vi "Translator.Translate.Controls.vi"(7 "group":string, 8 "error in":errorcluster, 9 "font name":string, 10 "Controls out":T1[](array[typedef]), 11 "Translation file":path=path "D:/PL_0125_Sapphire_Automation_branches/SOFTWARE_v1.1-Translation/settings/Translation-Chinese.ini") -> (0 "error out":errorcluster)   [LabVIEW 2019, in "Tools.lvlib"]
uses:
  Tools.lvlib
  Translator.ControlData.ctl
  Translator.ControlTypes.ctl
  <vilib>/Utility/miscctls.llb/LVRowAndColumnTypeDef.ctl
  Translator.File.MatchStrings (Single).vi
  Translator.File.MatchStrings (Array).vi
  <vilib>/Utility/config.llb/NI_LVConfig.lvlib
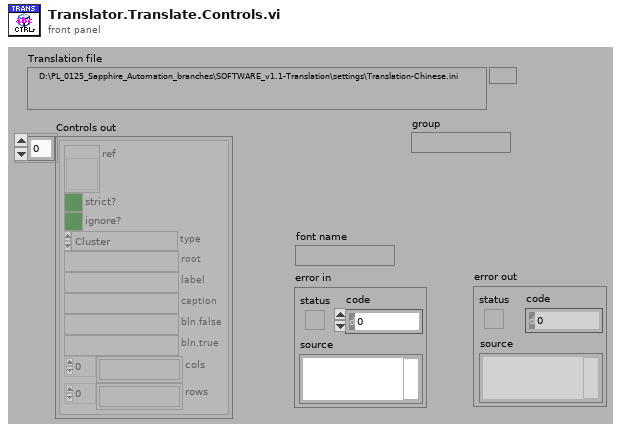
[diagram p1: front panel]
types:
  T1 = typedef "Tools.lvlib/Translator.ControlData.ctl" = cluster{"ref":refnum<vi>, "strict?":bool, "ignore?":bool, "type":T2, "root":string, "label":string, "caption":string, "bln.false":string, "bln.true":string, "cols":string[], "rows":string[]}
  T2 = typedef "Tools.lvlib/Translator.ControlTypes.ctl" = enum16{"Cluster", "Array", "Boolean", "Ring", "String", "Tab", "Listbox", "Multicolumn listbox", "Table", "Other"}
  T3 = typedef "LVRowAndColumnTypeDef.ctl" = cluster{"Row":i32, "Column":i32}
  T4 = typedef "NI_LVConfig.lvlib/Config Data RefNum.ctl" = refnum<k1>
  T5 = typedef "LVBoundsTypeDef.ctl" = cluster{"Width":u32, "Height":u32}
  T6 = typedef "LVPositionTypeDef.ctl" = cluster{"Left":i32, "Top":i32}
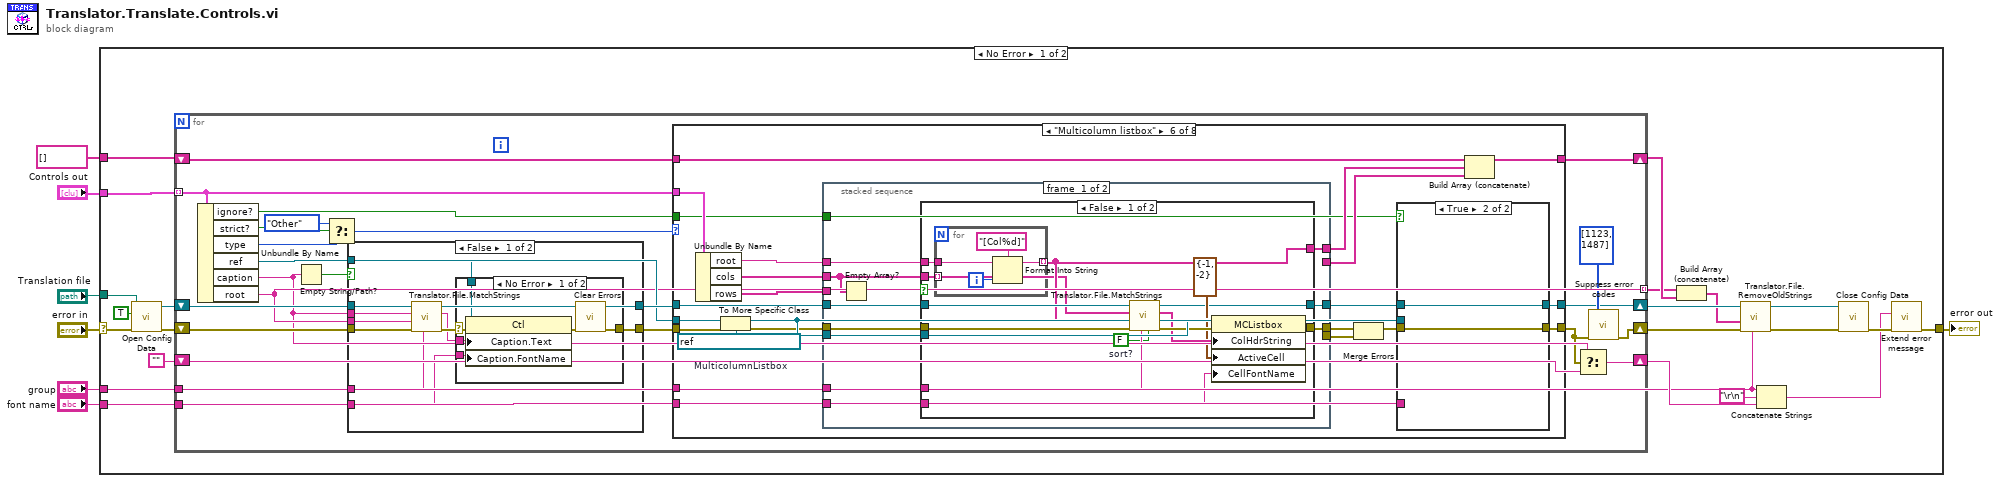
[diagram p0: block diagram]
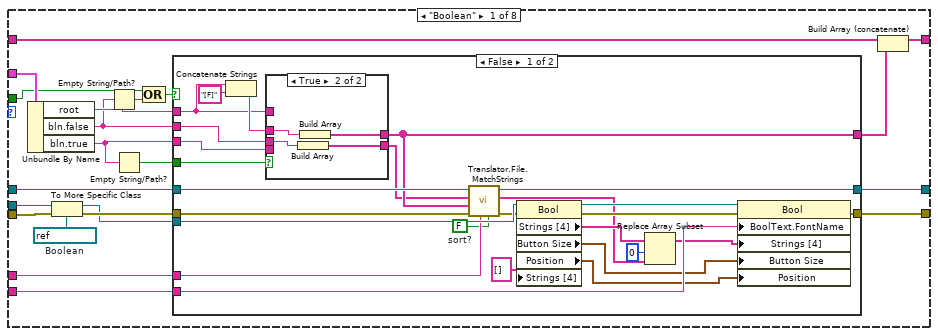
[diagram p4: hidden frame]
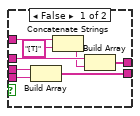
[diagram p5: hidden frame]
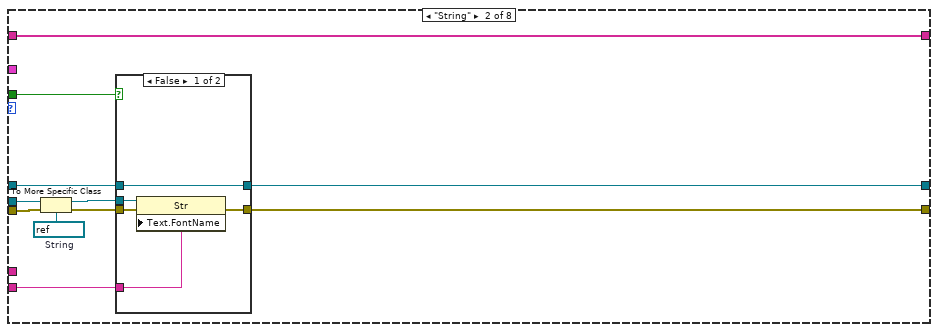
[diagram p7: hidden frame]
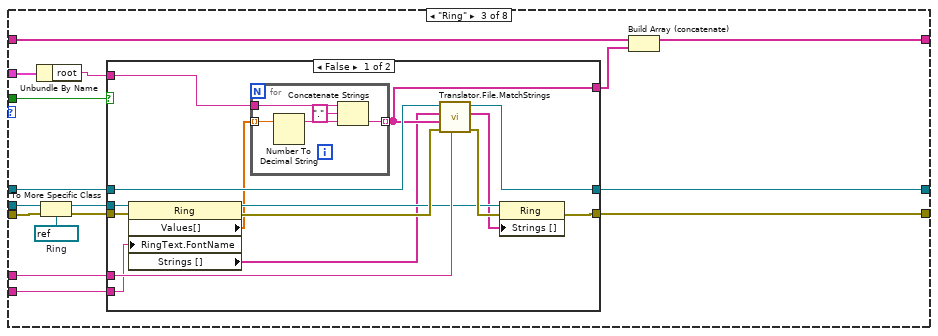
[diagram p9: hidden frame]
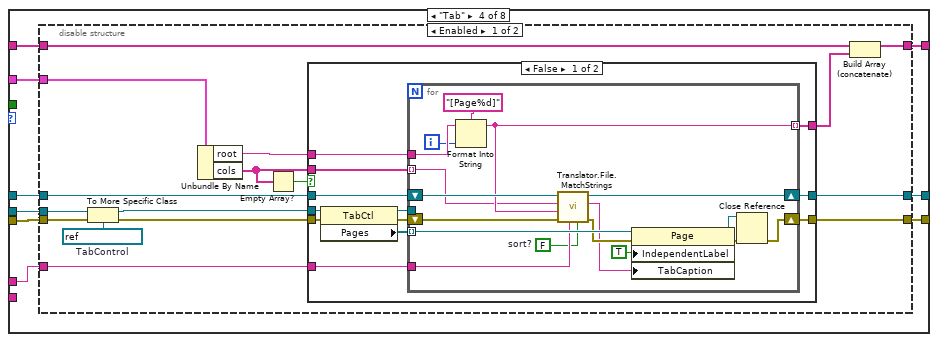
[diagram p11: hidden frame]
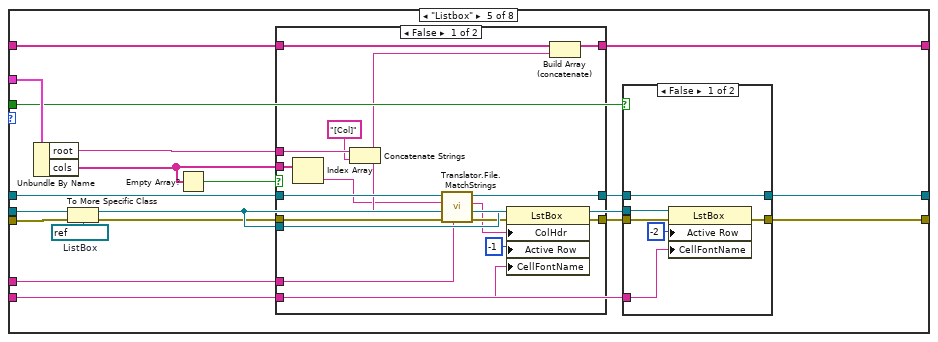
[diagram p14: hidden frame]
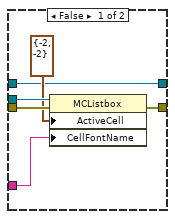
[diagram p17: hidden frame]
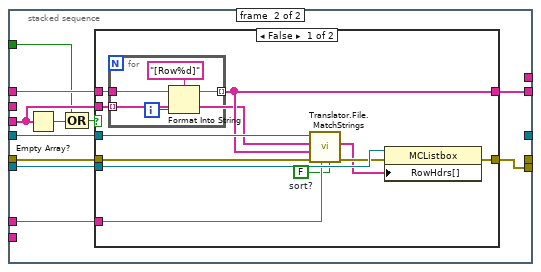
[diagram p19: hidden frame]
diagram:
  n1 = case shown="No Error" "error in" {
    selector: "error in" -> [w17 w477]
    tunnel: "Controls out" -> [w22 _]
    tunnel: [w15 w477] -> w5
    tunnel: "Translation file" -> [w11 _]
    tunnel: "group" -> [w10 _]
    tunnel: "font name" -> [w29 _]
    tunnel: string[] [] -> [w26 _]
    frame No Error {
      n2 = call <vilib>:"Open Config Data.vi"("error in (no error)"=w17, "create file if necessary (T)"=TRUE, "configuration file path"=w11) -> ("error out"=w8:errorcluster, "refnum"=w9:T4)  [unwired: 6 in, 1 out]
      n3 = for {
        tunnel: w22 -> [w53] mode=indexing
        tunnel: w10 -> [w50]
        shift-right: [w30] -> w28
        shift-left: w9 -> [w51]
        tunnel: w29 -> [w31]
        shift-right: [w40] -> w25
        shift-left: w26 -> [w41]
        tunnel: [w39] -> w24 mode=indexing
        shift-right: [w35] -> w20
        shift-left: "" -> [w37]
        shift-right: [w33] -> w27
        shift-left: w8 -> [w52]
        n4 = Unbundle By Name(w53) -> ("ignore?"=w38:bool, "strict?"=w45:bool, "type"=w44:T2, "ref"=w46:refnum<vi>, "caption"=w36:string, "root"=w39:string)
        n5 = Empty String/Path?(string/path=w36) -> (empty?=w47:bool)
        n6 = Select(t=Translator.ControlTypes."Other", s=w45, f=w44) -> (s? t:f=w42:T2)
        n7 = case shown="False" w47 {
          tunnel: w52 -> [w55 w72]
          tunnel: w51 -> [w63 w71]
          tunnel: w50 -> [w56 _]
          tunnel: [w62 w71] -> w49
          tunnel: [w61 w72] -> w48
          tunnel: w46 -> [w60 _]
          tunnel: w31 -> [w58 _]
          tunnel: w36 -> [w54 _]
          tunnel: w39 -> [w57 _]
          frame False {
            n8 = call-poly "Translator.File.MatchStrings.vi"("group"=w56, "error in"=w55, "label"=w57, "default value"=w54, "refnum in"=w63) -> ("error out"=w61:errorcluster, "value out"=w59:string, "refnum out"=w62:T4)  [unwired: 3 in, 1 out]
            n9 = case shown="No Error" w61 {
              selector: w61 -> [w69 w70]
              tunnel: [w65 w70] -> _
              tunnel: w60 -> [w67 _]
              tunnel: w58 -> [w66 _]
              tunnel: w59 -> [w64 _]
              frame No Error {
                n10 = property class="Ctl"(reference=w67, error in=w69, "Caption.Text"=w64, "Caption.FontName"=w66) -> (error out=w68:errorcluster)  [unwired: 1 out]
                n11 = call <vilib>:"Clear Errors.vi"("error in (no error)"=w68) -> ("error out"=w65:errorcluster)  [unwired: 5 in, 1 out]
              }
              frame Error {
              }
            }
          }
          frame True {
          }
        }
        n12 = case shown="\"Multicolumn listbox\"" w42 {
          tunnel: w46 -> [w91 w142 w165 w197 w261 w308 w397 _]
          tunnel: w48 -> [w92 w143 w166 w198 w262 w309 w398 w476]
          tunnel: w53 -> [w90 _ w154 w191 w266 w316 w405 _]
          tunnel: [w76 w138 w161 w196 w256 w305 w395 w476] -> w34
          tunnel: w49 -> [w88 w134 w158 w195 w264 w314 w403 w474]
          tunnel: w50 -> [w89 _ w157 w194 w263 w312 w401 _]
          tunnel: w31 -> [w74 w139 w162 _ w250 w297 w386 _]
          tunnel: w41 -> [w84 w137 w160 w193 w254 w301 w392 w475]
          tunnel: [w86 w137 w155 w192 w253 w302 w389 w475] -> w40
          tunnel: w38 -> [w75 w136 w159 _ w252 w298 w387 _]
          tunnel: [w73 w135 w156 w190 w249 w296 w385 w474] -> w30
          frame "Boolean" {
            w93 = refnum<vi> refnum  # Boolean
            n13 = Unbundle By Name(w90) -> ("root"=w87:string, "bln.false"=w83:string, "bln.true"=w82:string)
            n14 = To More Specific Class(target class=w93, reference=w91, error in=w92) -> (specific class reference=w77:refnum<vi>, error out=w80:errorcluster)
            n15 = Empty String/Path?(string/path=w83) -> (empty?=w79:bool)
            n16 = Empty String/Path?(string/path=w82) -> (empty?=w81:bool)
            n17 = Compound Arithmetic op=OR(w75, w79) -> (w78:bool)
            n18 = case shown="False" w78 {
              tunnel: w77 -> [w113 _]
              tunnel: w80 -> [w98 w133]
              tunnel: [w119 w133] -> w76
              tunnel: w87 -> [w108 _]
              tunnel: w89 -> [w99 _]
              tunnel: w88 -> [w111 w132]
              tunnel: [w100 _] -> w85
              tunnel: w82 -> [w106 _]
              tunnel: w83 -> [w107 _]
              tunnel: w81 -> [w110 _]
              tunnel: w74 -> [w105 _]
              tunnel: [w95 w132] -> w73
              frame False {
                w94 = FALSE  # sort?
                n19 = Concatenate Strings(w108, "[F]" ("format string")) -> (w109:string)
                n20 = case shown="True" w110 {
                  tunnel: w108 -> [w126 _]
                  tunnel: [w125 w130] -> w100
                  tunnel: w109 -> [w124 w131]
                  tunnel: w107 -> [w122 w129]
                  tunnel: w106 -> [w121 _]
                  tunnel: [w120 w128] -> w97
                  frame False {
                    n21 = Build Array(w122, w121) -> (w120:string[])
                    n22 = Concatenate Strings(w126, "[T]" ("format string")) -> (w123:string)
                    n23 = Build Array(w124, w123) -> (w125:string[])
                  }
                  frame True {
                    n24 = Build Array(w129) -> (w128:string[])
                    n25 = Build Array(w131) -> (w130:string[])
                  }
                }
                n26 = call-poly "Translator.File.MatchStrings.vi"("sort? (T)"=w94, "group"=w99, "error in"=w98, "labels"=w100, "default values"=w97, "refnum in"=w111) -> ("error out"=w112:errorcluster, "values out"=w102:string[], "refnum out"=w95:T4)  [unwired: 2 in, 1 out]
                n27 = property class="Bool"(reference=w113, error in=w112, "Strings [4]"=string[] []) -> (reference out=w115:refnum<vi>, error out=w116:errorcluster, "Strings [4]"=w118:string[], "Button Size"=w103:T5, "Position"=w101:T6)
                n28 = Replace Array Subset(array=w118, new element=w102, index=0) -> (w104:string[])
                n29 = property class="Bool"(reference=w115, error in=w116, "BoolText.FontName"=w105, "Strings [4]"=w104, "Button Size"=w103, "Position"=w101) -> (error out=w119:errorcluster)  [unwired: 1 out]
              }
              frame True {
              }
            }
            n30 = Build Array (concatenate)(w84, w85) -> (w86:string[])
          }
          frame "String" {
            w144 = refnum<vi> refnum  # String
            n31 = To More Specific Class(target class=w144, reference=w142, error in=w143) -> (specific class reference=w141:refnum<vi>, error out=w140:errorcluster)
            n32 = case shown="False" w136 {
              tunnel: w141 -> [w149 _]
              tunnel: w140 -> [w148 w151]
              tunnel: w139 -> [w146 _]
              tunnel: [w147 w151] -> w138
              tunnel: [w145 w150] -> w135
              tunnel: w134 -> [w145 w150]
              frame False {
                n33 = property class="Str"(reference=w149, error in=w148, "Text.FontName"=w146) -> (error out=w147:errorcluster)  [unwired: 1 out]
              }
              frame True {
              }
            }
          }
          frame "Ring" {
            w167 = refnum<vi> refnum  # Ring
            n34 = Unbundle By Name(w154) -> ("root"=w153:string)
            n35 = To More Specific Class(target class=w167, reference=w165, error in=w166) -> (specific class reference=w164:refnum<vi>, error out=w163:errorcluster)
            n36 = case shown="False" w159 {
              tunnel: w164 -> [w182 _]
              tunnel: w163 -> [w181 w189]
              tunnel: w162 -> [w172 _]
              tunnel: [w176 w189] -> w161
              tunnel: w158 -> [w179 w188]
              tunnel: w157 -> [w178 _]
              tunnel: [w173 w188] -> w156
              tunnel: w153 -> [w170 _]
              tunnel: [w169 _] -> w152
              frame False {
                n37 = property class="Ring"(reference=w182, error in=w181, "RingText.FontName"=w172) -> (reference out=w175:refnum<vi>, error out=w180:errorcluster, "Values[]"=w171:ext[], "Strings []"=w168:string[])
                n38 = for {
                  tunnel: w171 -> [w184] mode=indexing
                  tunnel: [w186] -> w169 mode=indexing
                  tunnel: w170 -> [w185]
                  n39 = Number To Decimal String(number=w184) -> (decimal integer string=w183:string)  [unwired: 1 in]
                  n40 = Concatenate Strings(w185, "." ("string"), w183) -> (w186:string)
                }
                n41 = call-poly "Translator.File.MatchStrings.vi"("group"=w178, "error in"=w180, "labels"=w169, "default values"=w168, "refnum in"=w179) -> ("error out"=w177:errorcluster, "values out"=w174:string[], "refnum out"=w173:T4)  [unwired: 3 in, 1 out]
                n42 = property class="Ring"(reference=w175, error in=w177, "Strings []"=w174) -> (error out=w176:errorcluster)  [unwired: 1 out]
              }
              frame True {
              }
            }
            n43 = Build Array (concatenate)(w160, w152) -> (w155:string[])
          }
          frame "Tab" {
            n44 = disable-structure shown="Enabled" {
              disable-tunnel: w198 -> [w214 w246]
              disable-tunnel: w197 -> [w213 _]
              disable-tunnel: [w212 w246] -> w196
              disable-tunnel: w195 -> [w211 _]
              disable-tunnel: w194 -> [w210 _]
              disable-tunnel: w193 -> [w209 w247]
              disable-tunnel: [w208 w247] -> w192
              disable-tunnel: w191 -> [w200 _]
              disable-tunnel: [w199 _] -> w190
              frame Enabled {
                w205 = refnum<vi> refnum  # TabControl
                n45 = To More Specific Class(target class=w205, reference=w213, error in=w214) -> (specific class reference=w206:refnum<vi>, error out=w207:errorcluster)
                n46 = Unbundle By Name(w200) -> ("root"=w204:string, "cols"=w203:string[])
                n47 = Empty Array?(array=w203) -> (empty?=w202:bool)
                n48 = case shown="False" w202 {
                  tunnel: w207 -> [w225 w245]
                  tunnel: w206 -> [w222 _]
                  tunnel: [w221 w245] -> w212
                  tunnel: w211 -> [w220 w244]
                  tunnel: w204 -> [w219 _]
                  tunnel: w203 -> [w218 _]
                  tunnel: w210 -> [w217 _]
                  tunnel: [w216 _] -> w201
                  tunnel: [w215 w244] -> w199
                  frame False {
                    n49 = property class="TabCtl"(reference=w222, error in=w225) -> (reference out=w223:refnum<vi>, error out=w224:errorcluster, "Pages"=w226:refnum<vi>[])
                    n50 = for {
                      tunnel: w226 -> [w243] mode=indexing
                      tunnel: w223 -> [_]
                      shift-right: [w239] -> w221
                      shift-left: w224 -> [w229]
                      tunnel: w218 -> [w230] mode=indexing
                      tunnel: w219 -> [w238]
                      tunnel: w217 -> [w232]
                      tunnel: [w231] -> w216 mode=indexing
                      shift-right: [w228] -> w215
                      shift-left: w220 -> [w241]
                      i -> [w236]
                      w227 = FALSE  # sort?
                      n51 = Format Into String(format string="[Page%d]", initial string=w238, w236) -> (resulting string=w231:string)  [unwired: 1 in, 1 out]
                      n52 = call-poly "Translator.File.MatchStrings.vi"("sort? (F)"=w227, "group"=w232, "error in"=w229, "label"=w231, "default value"=w230, "refnum in"=w241) -> ("error out"=w242:errorcluster, "value out"=w235:string, "refnum out"=w228:T4)  [unwired: 2 in, 1 out]
                      n53 = property class="Page"(reference=w243, error in=w242, "IndependentLabel"=TRUE ("Independent Label"), "TabCaption"=w235) -> (reference out=w234:refnum<vi>, error out=w240:errorcluster)
                      n54 = Close Reference(reference=w234, error in (no error)=w240) -> (error out=w239:errorcluster)
                    }
                  }
                  frame True {
                  }
                }
                n55 = Build Array (concatenate)(w209, w201) -> (w208:string[])
              }
              frame Disabled {
              }
            }
          }
          frame "Listbox" {
            w260 = refnum<vi> refnum  # ListBox
            n56 = Unbundle By Name(w266) -> ("root"=w265:string, "cols"=w259:string[])
            n57 = To More Specific Class(target class=w260, reference=w261, error in=w262) -> (specific class reference=w258:refnum<vi>, error out=w255:errorcluster)
            n58 = Empty Array?(array=w259) -> (empty?=w251:bool)
            n59 = case shown="False" w251 {
              tunnel: [w291 w294] -> w257
              tunnel: w255 -> [w276 w294]
              tunnel: w265 -> [w290 _]
              tunnel: w259 -> [w285 _]
              tunnel: w264 -> [w289 w292]
              tunnel: w263 -> [w278 _]
              tunnel: w258 -> [w288 _]
              tunnel: w254 -> [w283 w293]
              tunnel: [w282 w293] -> w253
              tunnel: w250 -> [w280 _]
              tunnel: [w275 w292] -> w248
              frame False {
                n60 = Index Array(array=w285) -> (element=w277:string)  [unwired: 1 in]
                n61 = Concatenate Strings(w290, "[Col]" ("format string")) -> (w279:string)
                n62 = call-poly "Translator.File.MatchStrings.vi"("group"=w278, "error in"=w276, "label"=w279, "default value"=w277, "refnum in"=w289) -> ("error out"=w287:errorcluster, "value out"=w284:string, "refnum out"=w275:T4)  [unwired: 3 in, 1 out]
                n63 = property class="LstBox"(reference=w288, error in=w287, "ColHdr"=w284, "Active Row"=-1 ("Active Row:Active Row Number"), "CellFontName"=w280) -> (error out=w291:errorcluster)  [unwired: 1 out]
                n64 = Build Array (concatenate)(w283, w279) -> (w282:string[])
              }
              frame True {
              }
            }
            n65 = case shown="False" w252 {
              tunnel: w258 -> [w272 _]
              tunnel: w257 -> [w271 w274]
              tunnel: w250 -> [w269 _]
              tunnel: [w268 w274] -> w256
              tunnel: [w267 w273] -> w249
              tunnel: w248 -> [w267 w273]
              frame False {
                n66 = property class="LstBox"(reference=w272, error in=w271, "Active Row"=-2 ("Active Row:Active Row Number"), "CellFontName"=w269) -> (error out=w268:errorcluster)  [unwired: 1 out]
              }
              frame True {
              }
            }
          }
          frame "Multicolumn listbox" {
            w307 = refnum<vi> refnum  # MulticolumnListbox
            n67 = Unbundle By Name(w316) -> ("root"=w315:string, "cols"=w313:string[], "rows"=w311:string[])
            n68 = To More Specific Class(target class=w307, reference=w308, error in=w309) -> (specific class reference=w304:refnum<vi>, error out=w303:errorcluster)
            n69 = stacked-sequence {
              tunnel: [w330 _] -> w317
              tunnel: w303 -> [w336 w367]
              tunnel: w315 -> [w335 w366]
              tunnel: w314 -> [w334 w365]
              tunnel: w313 -> [w331 _]
              tunnel: w312 -> [w333 w364]
              tunnel: w311 -> [_ w363]
              tunnel: [_ w360] -> w310
              tunnel: w304 -> [w332 w362]
              tunnel: [w329 _] -> w300
              tunnel: [_ w361] -> w299
              tunnel: w298 -> [_ w357]
              tunnel: w297 -> [w328 _]
              tunnel: [w326 _] -> w295
              frame #0 {
                n70 = Empty Array?(array=w331) -> (empty?=w327:bool)
                n71 = case shown="False" w327 {
                  tunnel: [w350 w356] -> w330
                  tunnel: w336 -> [w340 w356]
                  tunnel: w335 -> [w349 _]
                  tunnel: w331 -> [w339 _]
                  tunnel: w334 -> [w348 w355]
                  tunnel: w333 -> [w342 _]
                  tunnel: w332 -> [w347 _]
                  tunnel: [w341 _] -> w329
                  tunnel: w328 -> [w343 _]
                  tunnel: [w338 w355] -> w326
                  frame False {
                    w337 = FALSE  # sort?
                    n72 = for {
                      tunnel: w349 -> [w353]
                      tunnel: [w351] -> w341 mode=indexing
                      tunnel: w339 -> [_] mode=indexing
                      i -> [w352]
                      n73 = Format Into String(format string="[Col%d]", initial string=w353, w352) -> (resulting string=w351:string)  [unwired: 1 in, 1 out]
                    }
                    n74 = call-poly "Translator.File.MatchStrings.vi"("sort? (T)"=w337, "group"=w342, "error in"=w340, "labels"=w341, "default values"=w339, "refnum in"=w348) -> ("error out"=w346:errorcluster, "values out"=w345:string[], "refnum out"=w338:T4)  [unwired: 2 in, 1 out]
                    n75 = property class="MCListbox"(reference=w347, error in=w346, "ColHdrString"=w345, "ActiveCell"=T3 {"Row"=-1, "Column"=-2} ("Active Cell:Active Cell"), "CellFontName"=w343) -> (error out=w350:errorcluster)  [unwired: 1 out]
                  }
                  frame True {
                  }
                }
              }
              frame #1 {
                n76 = Empty Array?(array=w363) -> (empty?=w359:bool)
                n77 = Compound Arithmetic op=OR(w357, w359) -> (w358:bool)
                n78 = case shown="False" w358 {
                  tunnel: [w378 w383] -> w360
                  tunnel: w367 -> [w369 w383]
                  tunnel: w366 -> [w377 _]
                  tunnel: w363 -> [w370 _]
                  tunnel: w365 -> [w376 _]
                  tunnel: w364 -> [w372 _]
                  tunnel: w362 -> [w375 _]
                  tunnel: [w371 _] -> w361
                  frame False {
                    w368 = FALSE  # sort?
                    n79 = for {
                      tunnel: w377 -> [w381]
                      tunnel: [w379] -> w371 mode=indexing
                      tunnel: w370 -> [_] mode=indexing
                      i -> [w380]
                      n80 = Format Into String(format string="[Row%d]", initial string=w381, w380) -> (resulting string=w379:string)  [unwired: 1 in, 1 out]
                    }
                    n81 = call-poly "Translator.File.MatchStrings.vi"("sort? (T)"=w368, "group"=w372, "error in"=w369, "labels"=w371, "default values"=w370, "refnum in"=w376) -> ("error out"=w374:errorcluster, "values out"=w373:string[])  [unwired: 2 in, 2 out]
                    n82 = property class="MCListbox"(reference=w375, error in=w374, "RowHdrs[]"=w373) -> (error out=w378:errorcluster)  [unwired: 1 out]
                  }
                  frame True {
                  }
                }
              }
            }
            n83 = Merge Errors(w317, w310) -> (w306:errorcluster)
            n84 = case shown="True" w298 {
              tunnel: w306 -> [w323 w325]
              tunnel: [w322 w325] -> w305
              tunnel: w304 -> [w321 _]
              tunnel: w297 -> [w319 _]
              tunnel: [w318 w324] -> w296
              tunnel: w295 -> [w318 w324]
              frame False {
                n85 = property class="MCListbox"(reference=w321, error in=w323, "ActiveCell"=T3 {"Row"=-2, "Column"=-2} ("Active Cell:Active Cell"), "CellFontName"=w319) -> (error out=w322:errorcluster)  [unwired: 1 out]
              }
              frame True {
              }
            }
            n86 = Build Array (concatenate)(w301, w300, w299) -> (w302:string[])
          }
          frame "Table" {
            w394 = refnum<vi> refnum  # Table
            n87 = Unbundle By Name(w405) -> ("root"=w404:string, "cols"=w402:string[], "rows"=w400:string[])
            n88 = To More Specific Class(target class=w394, reference=w397, error in=w398) -> (specific class reference=w388:refnum<vi>, error out=w393:errorcluster)
            n89 = stacked-sequence {
              tunnel: [w418 _] -> w406
              tunnel: w393 -> [w424 w454]
              tunnel: w404 -> [w423 w453]
              tunnel: w403 -> [w422 w452]
              tunnel: w402 -> [w419 _]
              tunnel: w401 -> [w421 w451]
              tunnel: w400 -> [_ w450]
              tunnel: [_ w448] -> w399
              tunnel: w388 -> [w420 w449]
              tunnel: [_ w447] -> w391
              tunnel: [w417 _] -> w390
              tunnel: w387 -> [_ w444]
              tunnel: w386 -> [w415 _]
              tunnel: [_ w443] -> w384
              frame #0 {
                n90 = Empty Array?(array=w419) -> (empty?=w416:bool)
                n91 = case shown="False" w416 {
                  tunnel: [w437 w442] -> w418
                  tunnel: w424 -> [w426 w442]
                  tunnel: w423 -> [w436 _]
                  tunnel: w419 -> [w427 _]
                  tunnel: w422 -> [w435 _]
                  tunnel: w421 -> [w429 _]
                  tunnel: w420 -> [w434 _]
                  tunnel: [w428 _] -> w417
                  tunnel: w415 -> [w430 _]
                  frame False {
                    w425 = FALSE  # sort?
                    n92 = for {
                      tunnel: w436 -> [w440]
                      tunnel: [w438] -> w428 mode=indexing
                      tunnel: w427 -> [_] mode=indexing
                      i -> [w439]
                      n93 = Format Into String(format string="[Col%d]", initial string=w440, w439) -> (resulting string=w438:string)  [unwired: 1 in, 1 out]
                    }
                    n94 = call-poly "Translator.File.MatchStrings.vi"("sort? (T)"=w425, "group"=w429, "error in"=w426, "labels"=w428, "default values"=w427, "refnum in"=w435) -> ("error out"=w433:errorcluster, "values out"=w432:string[])  [unwired: 2 in, 2 out]
                    n95 = property class="Tbl"(reference=w434, error in=w433, "Column Headers[]"=w432, "Active Cell"=T3 {"Row"=-1, "Column"=-2} ("Active Cell:Active Cell"), "CellFontName"=w430) -> (error out=w437:errorcluster)  [unwired: 1 out]
                  }
                  frame True {
                  }
                }
              }
              frame #1 {
                n96 = Empty Array?(array=w450) -> (empty?=w446:bool)
                n97 = Compound Arithmetic op=OR(w444, w446) -> (w445:bool)
                n98 = case shown="False" w445 {
                  tunnel: [w467 w473] -> w448
                  tunnel: w454 -> [w458 w473]
                  tunnel: w453 -> [w466 _]
                  tunnel: w450 -> [w457 _]
                  tunnel: w452 -> [w465 w472]
                  tunnel: w451 -> [w460 _]
                  tunnel: w449 -> [w464 _]
                  tunnel: [w461 _] -> w447
                  tunnel: [w456 w472] -> w443
                  frame False {
                    w455 = FALSE  # sort?
                    n99 = for {
                      tunnel: w466 -> [w470]
                      tunnel: [w468] -> w461 mode=indexing
                      tunnel: w457 -> [_] mode=indexing
                      tunnel: [w468] -> w459 mode=indexing
                      i -> [w469]
                      n100 = Format Into String(format string="[Row%d]", initial string=w470, w469) -> (resulting string=w468:string)  [unwired: 1 in, 1 out]
                    }
                    n101 = call-poly "Translator.File.MatchStrings.vi"("sort? (T)"=w455, "group"=w460, "error in"=w458, "labels"=w459, "default values"=w457, "refnum in"=w465) -> ("error out"=w463:errorcluster, "values out"=w462:string[], "refnum out"=w456:T4)  [unwired: 2 in, 1 out]
                    n102 = property class="Tbl"(reference=w464, error in=w463, "Row Headers[]"=w462) -> (error out=w467:errorcluster)  [unwired: 1 out]
                  }
                  frame True {
                  }
                }
              }
            }
            n103 = Merge Errors(w406, w399) -> (w396:errorcluster)
            n104 = case shown="True" w387 {
              tunnel: w396 -> [w412 w414]
              tunnel: [w411 w414] -> w395
              tunnel: w386 -> [w409 _]
              tunnel: w388 -> [w408 _]
              tunnel: [w407 w413] -> w385
              tunnel: w384 -> [w407 w413]
              frame False {
                n105 = property class="Tbl"(reference=w408, error in=w412, "Active Cell"=T3 {"Row"=-2, "Column"=-2} ("Active Cell:Active Cell"), "CellFontName"=w409) -> (error out=w411:errorcluster)  [unwired: 1 out]
              }
              frame True {
              }
            }
            n106 = Build Array (concatenate)(w392, w390, w391) -> (w389:string[])
          }
          frame Default {
          }
        }
        n107 = Select(t=w36, s=w34, f=w37) -> (s? t:f=w35:string)
        n108 = call "Suppress error codes.vi"("error in (no error)"=w34, "suppress codes([43])"=i32[] [1123, 1487]) -> ("error out"=w33:errorcluster)  [unwired: 8 in, 1 out]
      }
      n109 = Build Array (concatenate)(w24, w25) -> (w23:string[])
      n110 = call "Translator.File.RemoveOldStrings.vi"("group"=w10, "error in"=w27, "labels"=w23, "refnum in"=w28) -> ("error out"=w12:errorcluster, "refnum out"=w14:T4)  [unwired: 5 in, 1 out]
      n111 = Concatenate Strings(w10, "\r\n", w20) -> (w13:string)
      n112 = call <vilib>:"Close Config Data.vi"("error in (no error)"=w12, "refnum"=w14) -> ("error out"=w16:errorcluster)  [unwired: 8 in, 1 out]
      n113 = call "Extend error message.vi"("error in"=w16, "extra message part"=w13) -> ("error out"=w15:errorcluster)  [unwired: 9 in]
    }
    frame Error {
    }
  }
  "error out" <- w5
